vi "Do Main Action.vi"(8 "error in (no error)":errorcluster, 10 "AbstractData":refnum<class "AbstractData.lvclass">, 11 "AbstractCollector in":refnum<class "AbstractCollector.lvclass">) -> (0 "error out":errorcluster, 3 "AbstractCollector out":refnum<class "AbstractCollector.lvclass">)   [LabVIEW 2014, in "AbstractCollector.lvclass"]
uses:
  AbstractCollector.lvclass
  Model/Data/AbstractData/AbstractData.lvclass
  Interfaces/Pipelined Actor/Pipelined Actor.lvclass
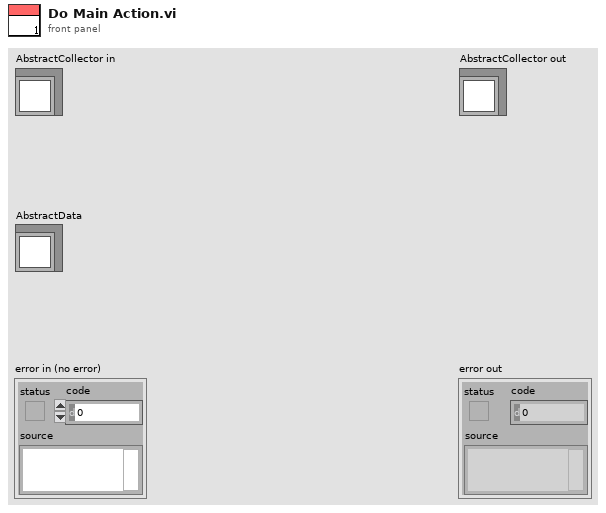
[diagram p1: front panel]
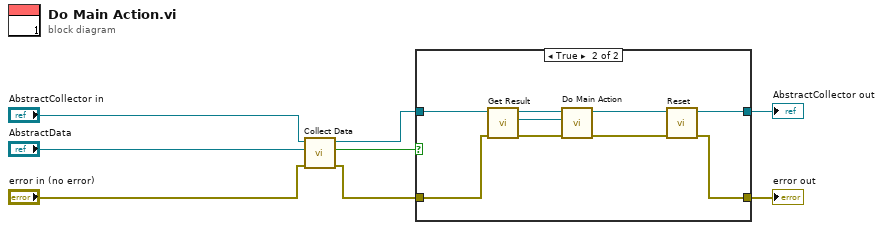
[diagram p0: block diagram]
diagram:
  n1 = call-dynamic "Collect Data.vi"("error in (no error)"="error in (no error)", "AbstractData in"="AbstractData", "AbstractCollector in"="AbstractCollector in") -> ("error out"=w1:errorcluster, "finished?"=w6:bool, "AbstractCollector out"=w3:refnum<class "AbstractCollector.lvclass">)  [unwired: 6 in]
  n2 = case shown="True" w6 {
    tunnel: [w9 w14] -> w8
    tunnel: w3 -> [w9 w11]
    tunnel: w1 -> [w10 w16]
    tunnel: [w10 w12] -> w7
    frame False {
    }
    frame True {
      n3 = call-dynamic "Get Result.vi"("error in (no error)"=w16, "AbstractCollector in"=w11) -> ("error out"=w17:errorcluster, "Collected Result out"=w18:refnum<class "AbstractData.lvclass">, "AbstractCollector out"=w19:refnum<class "AbstractCollector.lvclass">)  [unwired: 7 in]
      n4 = call-parent "Do Main Action.vi"("error in (no error)"=w17, "AbstractData"=w18, "Pipelined Actor in"=w19) -> ("error out"=w13:errorcluster, "Pipelined Actor out"=w15:refnum<class "AbstractCollector.lvclass">)  [unwired: 7 in]
      n5 = call-dynamic "Reset.vi"("error in (no error)"=w13, "AbstractCollector in"=w15) -> ("error out"=w12:errorcluster, "AbstractCollector out"=w14:refnum<class "AbstractCollector.lvclass">)  [unwired: 8 in]
    }
  }
  "error out" <- w7
  "AbstractCollector out" <- w8
